vi "TLCamera Main.vi"() -> ()   [LabVIEW 2020]
uses:
  Controls/Color Balance.ctl
  Controls/Region of Interest.ctl
  Controls/Binning.ctl
  Controls/Data Rate.ctl
  Controls/Taps.ctl
  Controls/Color Modes.ctl
  Controls/Trigger Settings.ctl
  Controls/Trigger Modes.ctl
  Controls/Trigger Polarity.ctl
  Status - Main.ctl
  SubVIs/Color/Color Processor References.ctl
  SubVIs/Parameters Get & Set/Get Parameters/Get ROIAndBin.vi
  SubVIs/Parameters Get & Set/Get Parameters/Get BinXRange.vi
  SubVIs/Parameters Get & Set/Get Parameters/Get BinYRange.vi
  SubVIs/Parameters Get & Set/Get Parameters/Get CameraSensorType.vi
  SubVIs/Parameters Get & Set/Get Parameters/Get BitDepth.vi
  SubVIs/Parameters Get & Set/Get Parameters/Get SensorHeight_pixels.vi
  SubVIs/Parameters Get & Set/Get Parameters/Get SensorWidth_pixels.vi
  SubVIs/Parameters Get & Set/Get Parameters/Get ExposureTimeRange_us.vi
  SubVIs/Parameters Get & Set/Set Parameters/Set ExposureTime_us.vi
  SubVIs/Parameters Get & Set/Get Parameters/Get GainRange.vi
  SubVIs/Parameters Get & Set/Set Parameters/Set Gain.vi
  SubVIs/Parameters Get & Set/Get Parameters/Get BlackLevelRange.vi
  SubVIs/Parameters Get & Set/Set Parameters/Set BlackLevel.vi
  SubVIs/Parameters Get & Set/Set Parameters/Set ROIAndBin.vi
  SubVIs/Parameters Get & Set/Set Parameters/Set FramesPerTrigger_zeroForUnlimited.vi
  SubVIs/Parameters Get & Set/Set Parameters/Set DataRate.vi
  SubVIs/Parameters Get & Set/Set Parameters/Set Taps.vi
  C:/code/Host/Installer/Scientific Camera Interfaces/LabVIEW/32_bit/Library_X86/Thorlabs.TSI.TLCameraInterfaces.dll
  code/Host/Installer/Scientific Camera Interfaces/LabVIEW/32_bit/Library_X86/Thorlabs.TSI.TLCameraInterfaces.dll
  C:/code/Host/Installer/Scientific Camera Interfaces/LabVIEW/32_bit/Library_X86/Thorlabs.TSI.Demosaicker.dll
  code/Host/Installer/Scientific Camera Interfaces/LabVIEW/32_bit/Library_X86/Thorlabs.TSI.Demosaicker.dll
  C:/code/Host/Installer/Scientific Camera Interfaces/LabVIEW/32_bit/Library_X86/Thorlabs.TSI.ColorProcessor.dll
  code/Host/Installer/Scientific Camera Interfaces/LabVIEW/32_bit/Library_X86/Thorlabs.TSI.ColorProcessor.dll
  C:/code/Host/Installer/Scientific Camera Interfaces/LabVIEW/32_bit/Library_X86/Thorlabs.TSI.ColorInterfaces.dll
  code/Host/Installer/Scientific Camera Interfaces/LabVIEW/32_bit/Library_X86/Thorlabs.TSI.ColorInterfaces.dll
panel:
  out "event callback refnum":refnum<k27>
  out "Status":T1
  in  "Exit":bool
  out "Frame Number":u32
  out "Camera Image":picture
  in  "Camera Settings":T11={"Color Balance"={"Red Gain"=1.0, "Green Gain"=1.0, "Blue Gain"=1.0}, "Region of Interest"={"Origin - X"=0, "Origin - Y"=0, "Width"=1392, "Height"=1040}, "Binning"={"Bin - X"=1, "Bin - Y"=1}, "Frame Settings"={"Frames per Trigger\n(zero for unlimited)"=0}, "Data Rate"={"DataRate"=enum."ReadoutSpeed20MHz", "Taps"=enum."SingleTap"}, "Image Type"=enum."Standard RGB", "Trigger Settings"={"Trigger Mode"=enum."Software", "Trigger Polarity"=enum."ActiveHigh"}, "Exposure (ms)"=100.0, "Gain"=0, "Black Level"=48} {"Black Level" max=100; "Gain" max=1023; "Binning"."Bin - Y" min=1 max=16; "Binning"."Bin - X" min=1 max=16; "Color Balance"."Blue Gain" min=0 max=10 step=0.05 scale=0.0..10.0 scale format="%#_3g"; "Color Balance"."Green Gain" min=0 max=10 step=0.05 scale=0.0..10.0 scale format="%#_3g"; "Color Balance"."Red Gain" min=0 max=10 step=0.05 scale=0.0..10.0 scale format="%#_3g"}
  in  "Close Camera":bool
  in  "Open Camera":bool
  in  "Stop Camera":bool
  in  "Start Camera":bool
  in  "Refresh":bool
  in  "Camera Serial Numbers":u16(ring) items=["ENG022"]
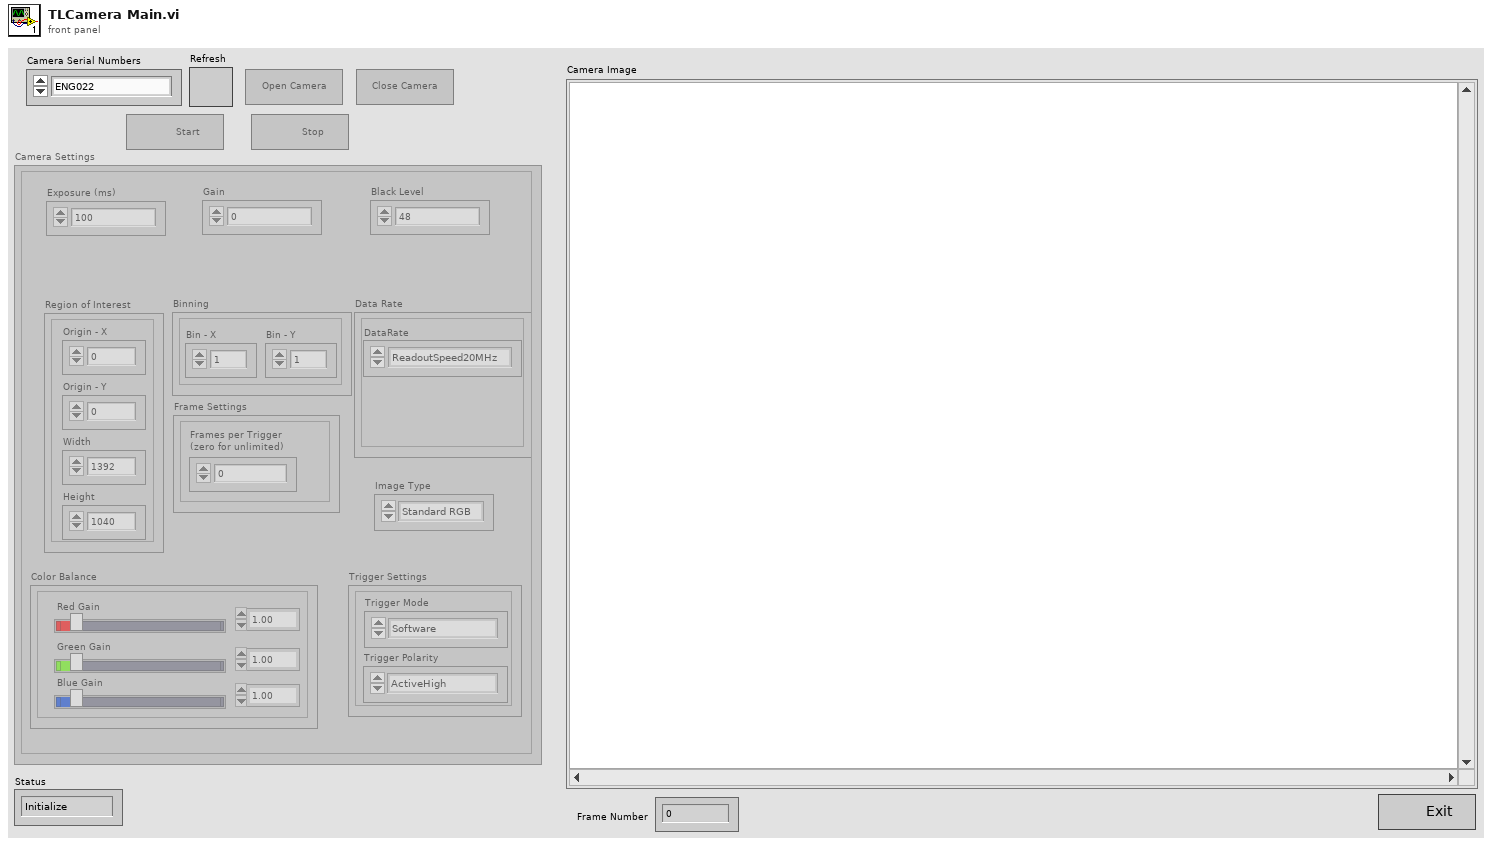
[diagram p1: front panel]
types:
  T1 = typedef "Status - Main.ctl" = enum16{"Initialize", "GUI", "Close"}
  T2 = typedef "Color Balance.ctl" = cluster{"Red Gain":sgl, "Green Gain":sgl, "Blue Gain":sgl}
  T3 = typedef "Region of Interest.ctl" = cluster{"Origin - X":u32, "Origin - Y":u32, "Width":u32, "Height":u32}
  T4 = typedef "Binning.ctl" = cluster{"Bin - X":u32, "Bin - Y":u32}
  T5 = typedef "Data Rate.ctl" = enum32{"ReadoutSpeed20MHz", "ReadoutSpeed40MHz", "FPS30", "FPS50"}
  T6 = typedef "Taps.ctl" = enum32{"SingleTap", "DualTap", "QuadTap"}
  T7 = typedef "Color Modes.ctl" = enum16{"Standard RGB", "Linear RGB", "Unprocessed"}
  T8 = typedef "Trigger Settings.ctl" = cluster{"Trigger Mode":T9, "Trigger Polarity":T10}
  T9 = typedef "Trigger Modes.ctl" = enum16{"Software", "Hardware Standard", "Bulb(PDX) Mode"}
  T10 = typedef "Trigger Polarity.ctl" = enum32{"ActiveHigh", "ActiveLow"}
  T11 = cluster{"Color Balance":T2, "Region of Interest":T3, "Binning":T4, "Frame Settings":cluster{"Frames per Trigger\n(zero for unlimited)":u32}, "Data Rate":cluster{"DataRate":T5, "Taps":T6}, "Image Type":T7, "Trigger Settings":T8, "Exposure (ms)":dbl, "Gain":u32, "Black Level":u32}
  T12 = typedef "Color Processor References.ctl" = cluster{"Demosaicker reference":refnum<k24>, "ColorProcessorSDK reference":refnum<k24>, "StandardRGBColorProcessor":refnum<k24>, "LinearRGBColorProcessor":refnum<k24>}
  T13 = enum8{"Enabled", "Disabled", "Disabled and Grayed Out"}
  T14 = cluster{"Thorlabs.TSI.TLCameraInterfaces.ITLCamera":refnum<k24>, "Frame Number":refnum<vi>, "Camera Image":refnum<vi>, "Value":T7, "Color Processor References":T12}
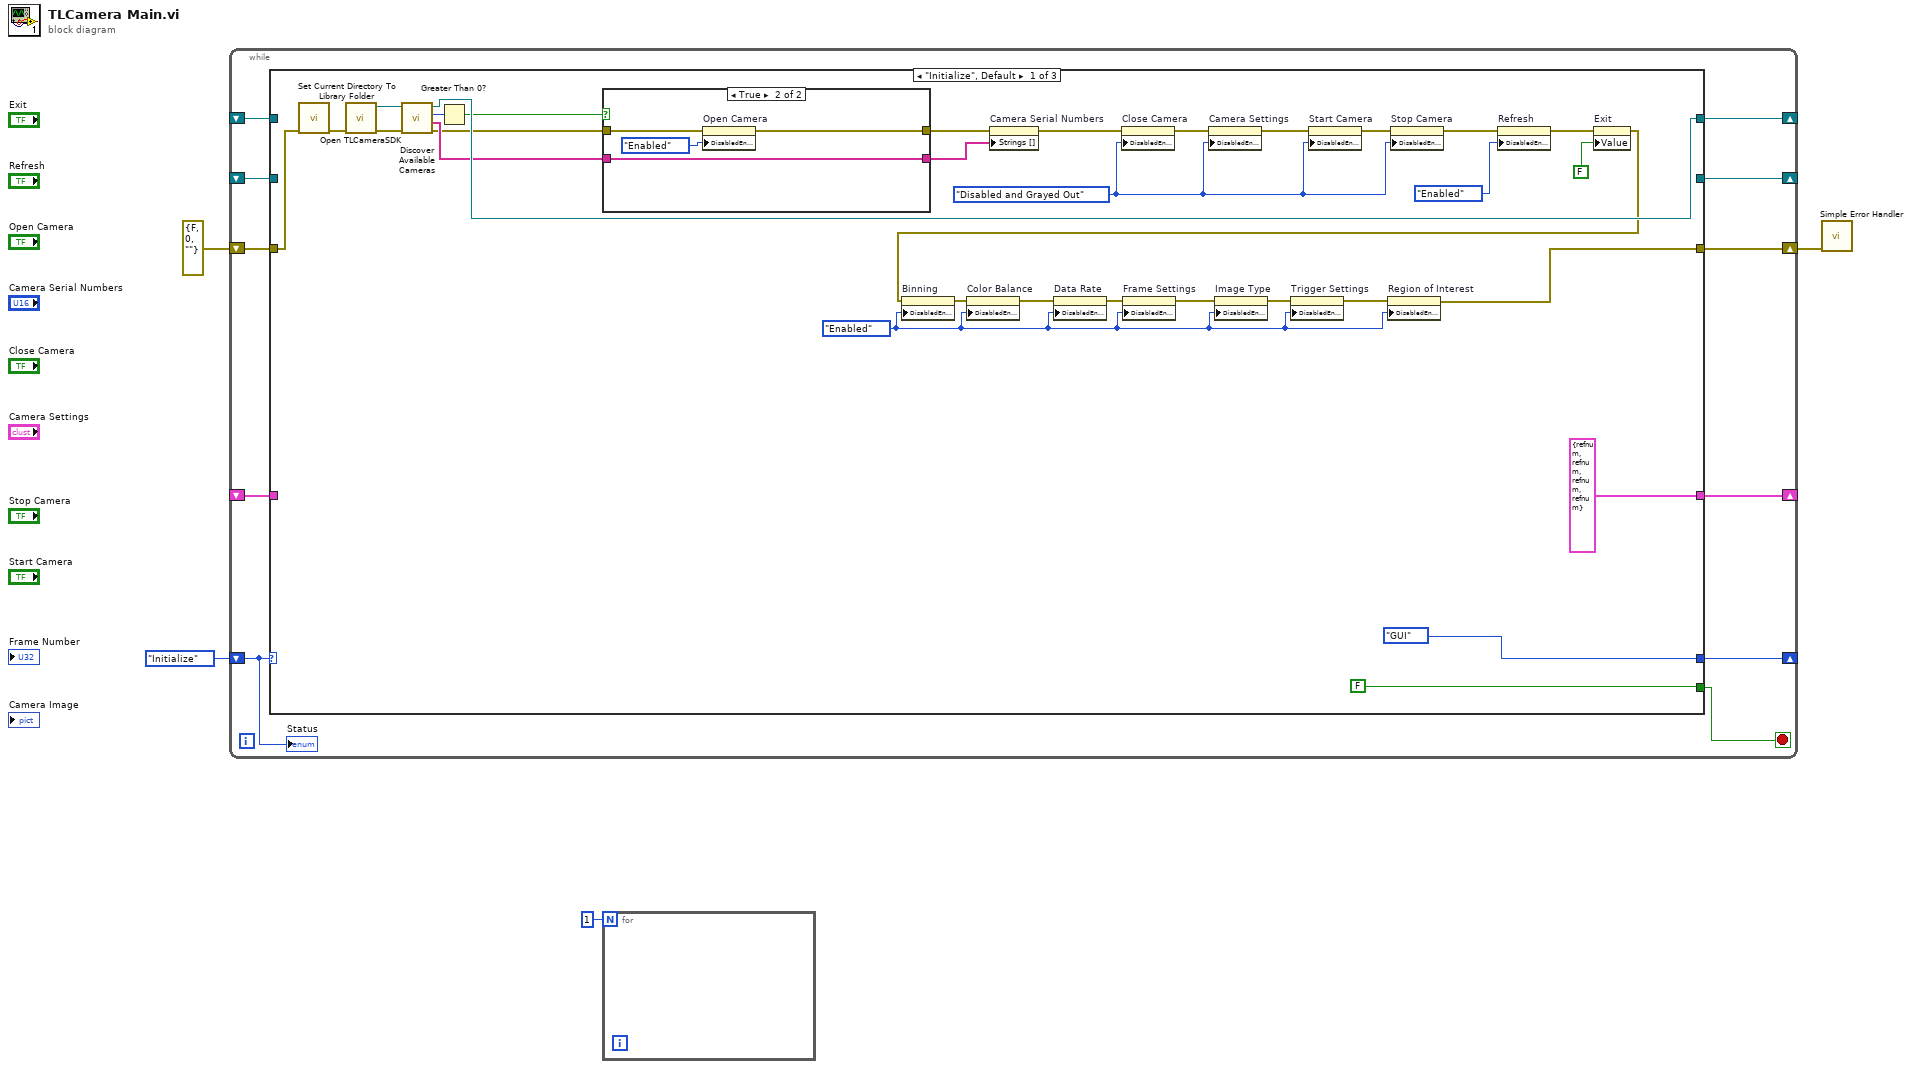
[diagram p0: block diagram]
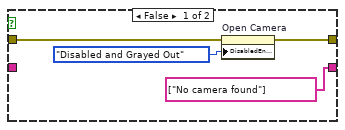
[diagram p2: hidden frame]
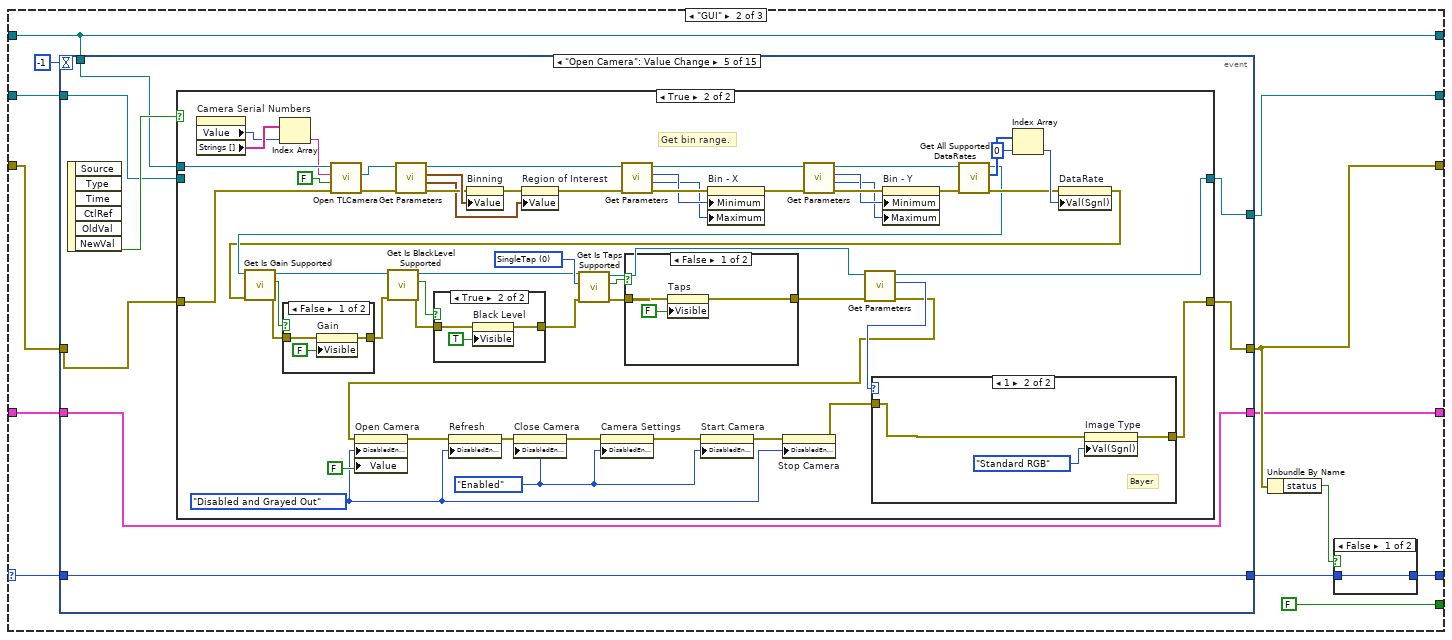
[diagram p3: hidden frame]
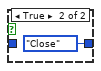
[diagram p4: hidden frame]
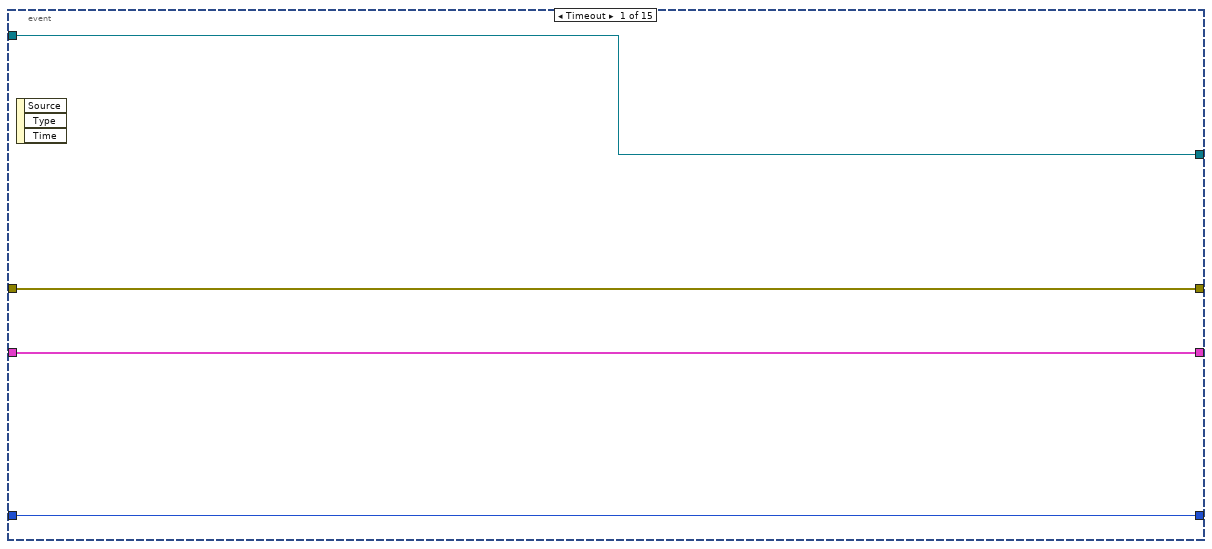
[diagram p5: hidden frame]
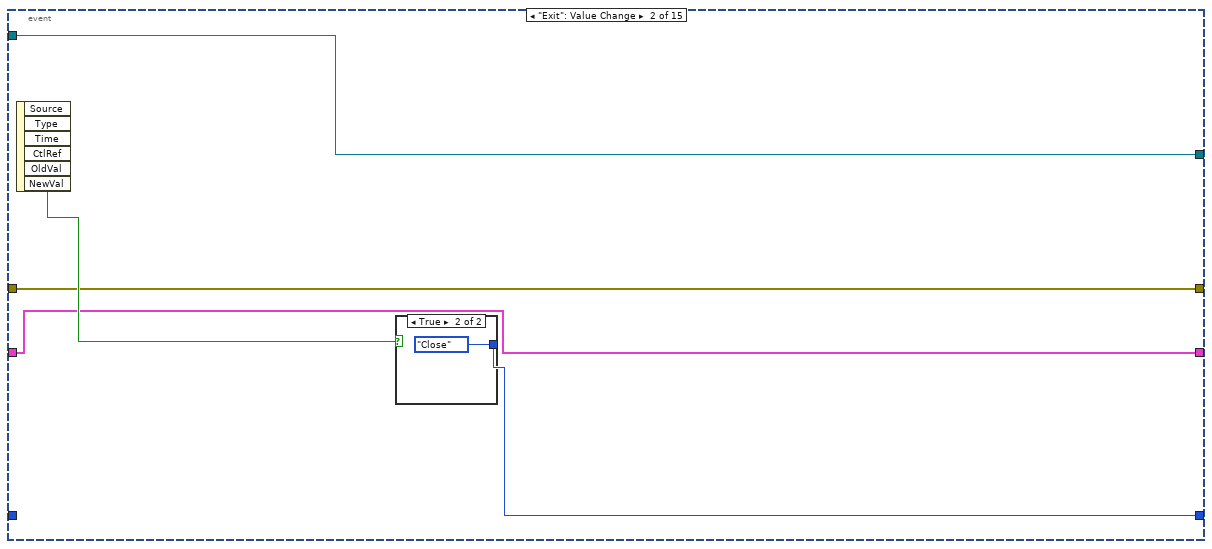
[diagram p6: hidden frame]
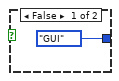
[diagram p7: hidden frame]
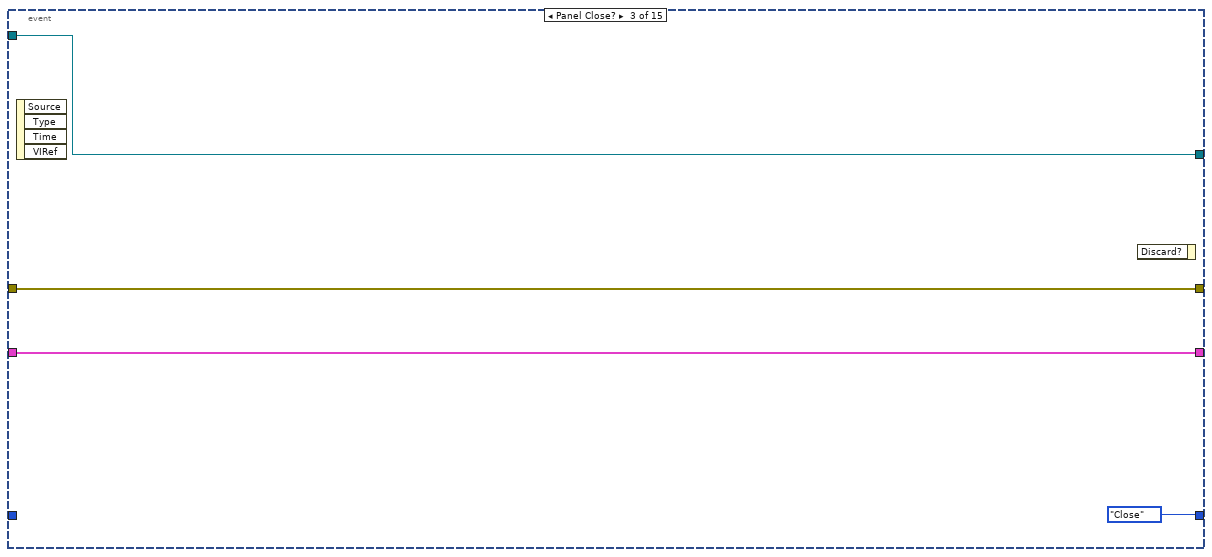
[diagram p8: hidden frame]
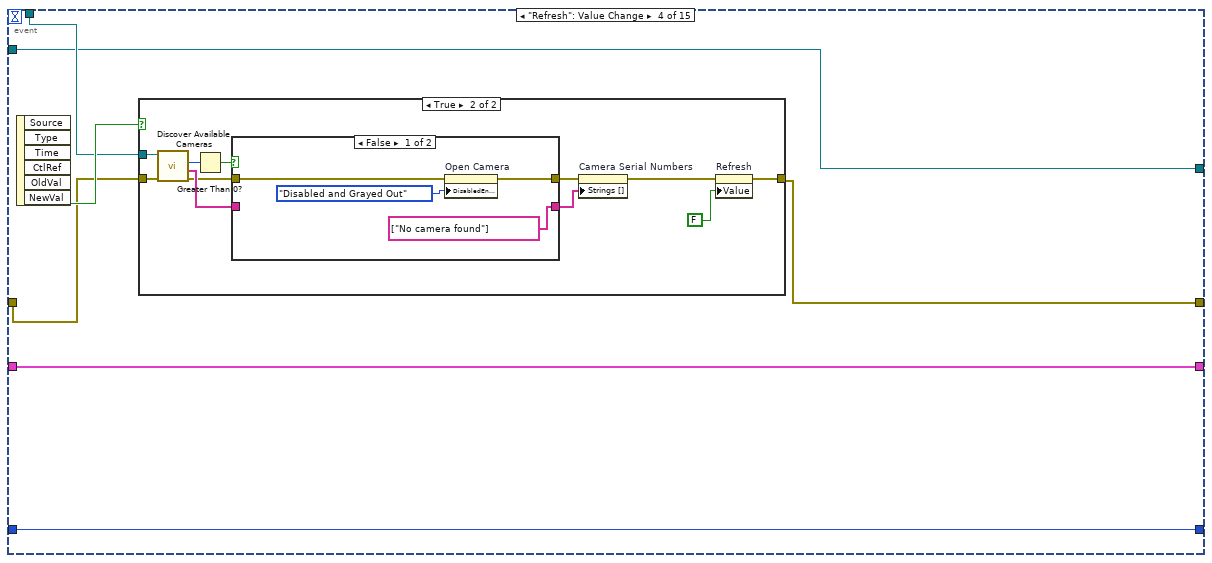
[diagram p9: hidden frame]
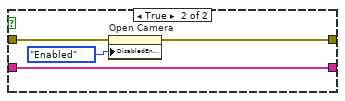
[diagram p11: hidden frame]
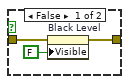
[diagram p13: hidden frame]
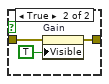
[diagram p14: hidden frame]
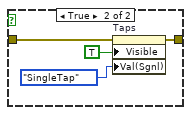
[diagram p15: hidden frame]
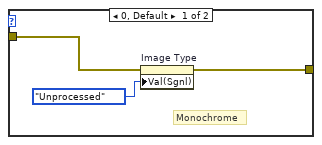
[diagram p16: hidden frame]
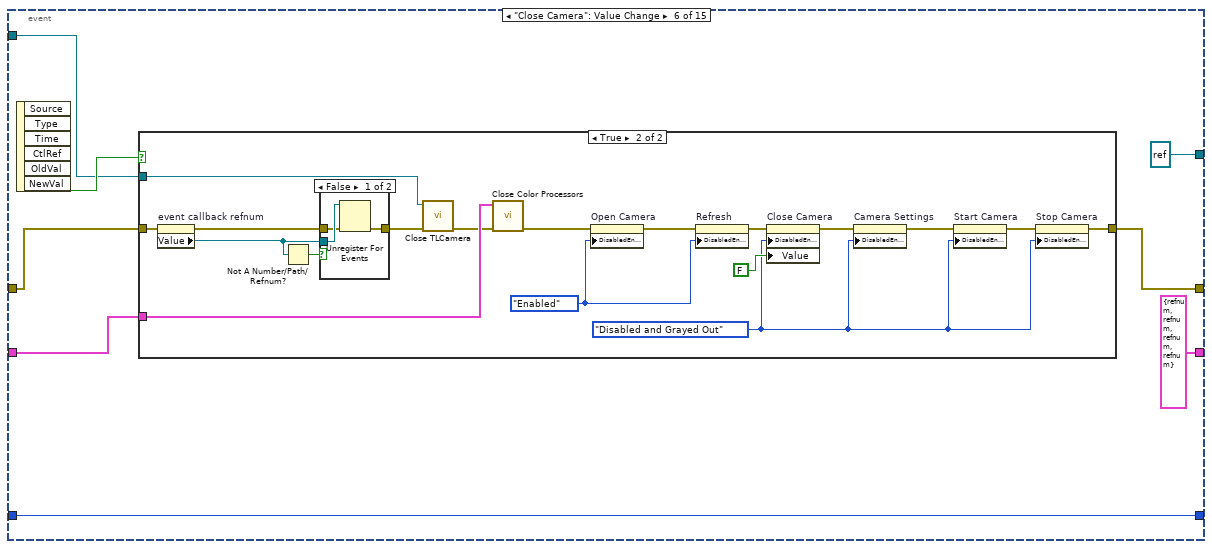
[diagram p17: hidden frame]
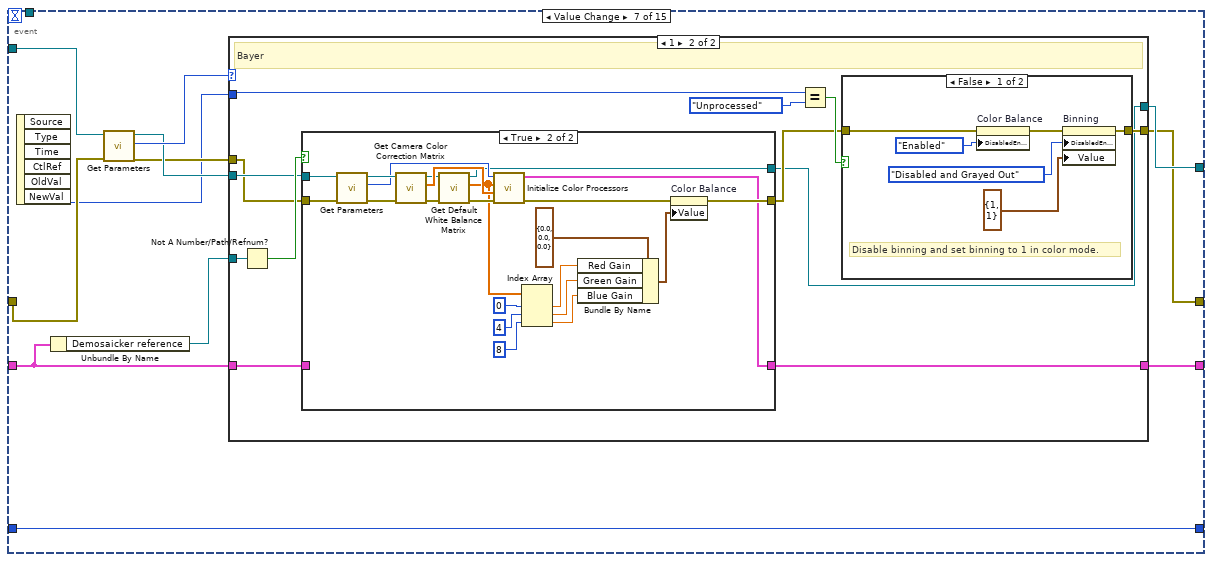
[diagram p20: hidden frame]
diagram:
  n1 = while {
    shift-right: [w8] -> _
    shift-left: Status_-_Main."Initialize" -> [w7]
    shift-right: [w15] -> _
    shift-left: _ -> [w14]
    shift-right: [w12] -> w2
    shift-left: errorcluster {"status"=FALSE, "code"=0, "source"=""} ("error in (no error)") -> [w13]
    shift-right: [w10] -> _
    shift-left: _ -> [w9]
    shift-right: [w5] -> _
    shift-left: _ -> [w6]
    stop <- w11 stop-if-true
    n2 = case shown="\"Initialize\", Default" w7 {
      selector: w7 -> [_ w66 w580]
      tunnel: [w46 w65 _] -> w15
      tunnel: w14 -> [_ w65 w582]
      tunnel: w13 -> [w18 w63 w563]
      tunnel: [w20 w62 w558] -> w12
      tunnel: [FALSE FALSE TRUE] -> w11
      tunnel: [Status_-_Main."GUI" w59 w580] -> w8
      tunnel: [_ w64 _] -> w10
      tunnel: w9 -> [_ w58 w577]
      tunnel: w6 -> [_ w57 w555]
      tunnel: [T12 {"Demosaicker reference"=refnum, "ColorProcessorSDK reference"=refnum, "StandardRGBColorProcessor"=refnum, "LinearRGBColorProcessor"=refnum} ("Color Processor References") w56 T12 {"Demosaicker reference"=refnum, "ColorProcessorSDK reference"=refnum, "StandardRGBColorProcessor"=refnum, "LinearRGBColorProcessor"=refnum} ("Color Processor References")] -> w5
      frame "Initialize", Default {
        w27 = T13."Enabled" ("Disabled")
        w36 = T13."Disabled and Grayed Out" ("Disabled")
        n3 = call "Set Current Directory To Library Folder.vi"("error in (no error)"=w18) -> ("error out"=w19:errorcluster)  [unwired: 10 in]
        n4 = call "Open TLCameraSDK.vi"("error in (no error)"=w19) -> ("error out"=w32:errorcluster, "Thorlabs.TSI.TLCameraInterfaces.ITLCameraSDK"=w31:refnum<k24>)  [unwired: 9 in]
        n5 = call "Discover Available Cameras.vi"("error in (no error)"=w32, "Thorlabs.TSI.TLCameraInterfaces.ITLCameraSDK"=w31) -> ("error out"=w42:errorcluster, "Serial Numbers"=w44:string[], "Number of Cameras"=w47:i32, "Thorlabs.TSI.TLCameraInterfaces.ITLCameraSDK"=w46:refnum<k24>)  [unwired: 6 in]
        n6 = Greater Than 0?(x=w47) -> (x > 0?=w45:bool)
        n7 = case shown="True" w45 {
          tunnel: w44 -> [_ w55]
          tunnel: [string[] ["No camera found"] ("Serial Numbers") w55] -> w43
          tunnel: w42 -> [w49 w53]
          tunnel: [w48 w52] -> w41
          frame False {
            n8 = property on="Open Camera" class="Bool (strict)"(error in=w49, "DisabledEnum"=T13."Disabled and Grayed Out" ("Disabled")) -> (error out=w48:errorcluster)  [unwired: 1 in, 1 out]
          }
          frame True {
            n9 = property on="Open Camera" class="Bool (strict)"(error in=w53, "DisabledEnum"=T13."Enabled" ("Disabled")) -> (error out=w52:errorcluster)  [unwired: 1 in, 1 out]
          }
        }
        n10 = property on="Camera Serial Numbers" class="Ring (strict)"(error in=w41, "Strings []"=w43) -> (error out=w40:errorcluster)  [unwired: 1 in, 1 out]
        n11 = property on="Close Camera" class="Bool (strict)"(error in=w40, "DisabledEnum"=w36) -> (error out=w39:errorcluster)  [unwired: 1 in, 1 out]
        n12 = property on="Camera Settings" class="Clust (strict)"(error in=w39, "DisabledEnum"=w36) -> (error out=w38:errorcluster)  [unwired: 1 in, 1 out]
        n13 = property on="Start Camera" class="Bool (strict)"(error in=w38, "DisabledEnum"=w36) -> (error out=w37:errorcluster)  [unwired: 1 in, 1 out]
        n14 = property on="Stop Camera" class="Bool (strict)"(error in=w37, "DisabledEnum"=w36) -> (error out=w30:errorcluster)  [unwired: 1 in, 1 out]
        n15 = property on="Refresh" class="Bool (strict)"(error in=w30, "DisabledEnum"=T13."Enabled" ("Disabled")) -> (error out=w29:errorcluster)  [unwired: 1 in, 1 out]
        n16 = property on="Exit" class="Bool (strict)"(error in=w29, "Value"=FALSE ("Camera Running")) -> (error out=w26:errorcluster)  [unwired: 1 in, 1 out]
        n17 = property on="Binning" class="Clust (strict)"(error in=w26, "DisabledEnum"=w27) -> (error out=w25:errorcluster)  [unwired: 1 in, 1 out]
        n18 = property on="Color Balance" class="Clust (strict)"(error in=w25, "DisabledEnum"=w27) -> (error out=w24:errorcluster)  [unwired: 1 in, 1 out]
        n19 = property on="Data Rate" class="Clust (strict)"(error in=w24, "DisabledEnum"=w27) -> (error out=w17:errorcluster)  [unwired: 1 in, 1 out]
        n20 = property on="Frame Settings" class="Clust (strict)"(error in=w17, "DisabledEnum"=w27) -> (error out=w23:errorcluster)  [unwired: 1 in, 1 out]
        n21 = property on="Image Type" class="Enum (strict)"(error in=w23, "DisabledEnum"=w27) -> (error out=w22:errorcluster)  [unwired: 1 in, 1 out]
        n22 = property on="Trigger Settings" class="Clust (strict)"(error in=w22, "DisabledEnum"=w27) -> (error out=w21:errorcluster)  [unwired: 1 in, 1 out]
        n23 = property on="Region of Interest" class="Clust (strict)"(error in=w21, "DisabledEnum"=w27) -> (error out=w20:errorcluster)  [unwired: 1 in, 1 out]
      }
      frame "GUI" {
        n24 = event shown="[4] \"Open Camera\": Value Change" {
          selector: _ -> [_ _ _ _ _ _ _ _ _ _ _ _ _ _ _]
          dyn-events: _ -> [_ _ _ _ _ _ _ _ _ _ _ _ _ _ _]
          timeout: -1 -> [_ _ _ _ _ _ _ _ _ _ _ _ _ _ _]
          tunnel: [w74 w78 Status_-_Main."Close" w88 w118 w207 w246 w317 w329 w348 w365 w396 w423 w488 w526] -> w60
          tunnel: w66 -> [w74 _ _ w88 w118 w207 w246 w317 w329 w348 w365 w396 w423 w488 w526]
          tunnel: w65 -> [_ _ _ w91 w119 _ _ _ _ _ _ _ _ _ _]
          tunnel: w63 -> [w73 w77 w84 w90 w117 w210 w245 w316 w332 w344 w367 w384 w421 w427 w529]
          tunnel: [w72 w76 w83 w87 w116 refnum<k24> refnum ("TLCamera reference") w240 w308 w320 w337 w357 w379 w424 w475 w528] -> w64
          tunnel: [w73 w77 w84 w89 w115 w209 w239 w309 w319 w336 w358 w380 w425 w472 w527] -> w62
          tunnel: w58 -> [w72 w76 w83 w87 w114 w206 w238 w307 w328 w343 w368 w379 w422 w473 w525]
          tunnel: w57 -> [w71 w75 w82 w86 w113 w204 w235 w305 w318 w334 w356 w378 w419 w438 w523]
          tunnel: [w71 w75 w82 w86 w113 T12 {"Demosaicker reference"=refnum, "ColorProcessorSDK reference"=refnum, "StandardRGBColorProcessor"=refnum, "LinearRGBColorProcessor"=refnum} ("Color Processor References") w236 w305 w318 w334 w356 w378 w419 w438 w523] -> w56
          event Timeout {
            n25 = event-data() -> ()  [unwired: 1 in, 3 out]
          }
          event "Exit": Value Change {
            n26 = event-data() -> ("NewVal"=w79:bool)  [unwired: 1 in, 5 out]
            n27 = case shown="True" w79 {
              tunnel: [Status_-_Main."GUI" Status_-_Main."Close"] -> w78
              frame False {
              }
              frame True {
              }
            }
          }
          event Panel Close? {
            n28 = event-data() -> ()  [unwired: 1 in, 4 out]
            n29 = event-data() -> ()  [unwired: 2 in, 1 out]
          }
          event "Refresh": Value Change {
            n30 = event-data() -> ("NewVal"=w92:bool)  [unwired: 1 in, 5 out]
            n31 = case shown="True" w92 {
              tunnel: w91 -> [_ w104]
              tunnel: w90 -> [w93 w103]
              tunnel: [w93 w94] -> w89
              frame False {
              }
              frame True {
                n32 = call "Discover Available Cameras.vi"("error in (no error)"=w103, "Thorlabs.TSI.TLCameraInterfaces.ITLCameraSDK"=w104) -> ("error out"=w100:errorcluster, "Serial Numbers"=w101:string[], "Number of Cameras"=w102:i32)  [unwired: 6 in, 1 out]
                n33 = Greater Than 0?(x=w102) -> (x > 0?=w97:bool)
                n34 = case shown="False" w97 {
                  tunnel: w101 -> [_ w112]
                  tunnel: [string[] ["No camera found"] ("Serial Numbers") w112] -> w99
                  tunnel: w100 -> [w106 w110]
                  tunnel: [w105 w109] -> w98
                  frame False {
                    n35 = property on="Open Camera" class="Bool (strict)"(error in=w106, "DisabledEnum"=T13."Disabled and Grayed Out" ("Disabled")) -> (error out=w105:errorcluster)  [unwired: 1 in, 1 out]
                  }
                  frame True {
                    n36 = property on="Open Camera" class="Bool (strict)"(error in=w110, "DisabledEnum"=T13."Enabled" ("Disabled")) -> (error out=w109:errorcluster)  [unwired: 1 in, 1 out]
                  }
                }
                n37 = property on="Camera Serial Numbers" class="Ring (strict)"(error in=w98, "Strings []"=w99) -> (error out=w95:errorcluster)  [unwired: 1 in, 1 out]
                n38 = property on="Refresh" class="Bool (strict)"(error in=w95, "Value"=FALSE ("Refresh")) -> (error out=w94:errorcluster)  [unwired: 1 in, 1 out]
              }
            }
          }
          event "Open Camera": Value Change {
            n39 = event-data() -> ("NewVal"=w120:bool)  [unwired: 1 in, 5 out]
            n40 = case shown="True" w120 {
              tunnel: w119 -> [_ w178]
              tunnel: w117 -> [w121 w146]
              tunnel: [w122 w124] -> w116
              tunnel: w114 -> [w122 _]
              tunnel: [w121 w147] -> w115
              frame False {
              }
              frame True {
                w145 = 0 items=["SingleTap", "DualTap", "QuadTap"] ("Taps")
                w165 = T13."Enabled" ("Disabled")
                w166 = T13."Disabled and Grayed Out" ("Disabled")
                # "Get bin range."
                n41 = property on="Camera Serial Numbers" class="Ring (strict)"() -> ("Value"=w176:u16, "Strings []"=w177:string[])  [unwired: 2 in, 2 out]
                n42 = Index Array(array=w177, index=w176) -> (element=w175:string)
                n43 = call "Open TLCamera.vi"("error in (no error)"=w146, "isDiagnosticsMessagesEnabled"=FALSE, "Camera serial number"=w175, "Thorlabs.TSI.TLCameraInterfaces.ITLCameraSDK"=w178) -> ("error out"=w163:errorcluster, "Thorlabs.TSI.TLCameraInterfaces.ITLCamera"=w162:refnum<k24>)  [unwired: 5 in, 1 out]
                n44 = call-poly "Get Parameters.vi"("error in (no error)"=w163, "Thorlabs.TSI.TLCameraInterfaces.ITLCamera"=w162) -> ("error out"=w160:errorcluster, "Region of Interest"=w159:T3, "Binning"=w161:T4, "Thorlabs.TSI.TLCameraInterfaces.ITLCamera"=w148:refnum<k24>)  [unwired: 6 in]
                n45 = property on="Binning" class="Clust (strict)"(error in=w160, "Value"=w161) -> (error out=w158:errorcluster)  [unwired: 1 in, 1 out]
                n46 = property on="Region of Interest" class="Clust (strict)"(error in=w158, "Value"=w159) -> (error out=w149:errorcluster)  [unwired: 1 in, 1 out]
                n47 = call-poly "Get Parameters.vi"("error in (no error)"=w149, "Thorlabs.TSI.TLCameraInterfaces.ITLCamera"=w148) -> ("error out"=w157:errorcluster, "Maximum"=w155:u32, "Minimum"=w156:u32, "Thorlabs.TSI.TLCameraInterfaces.ITLCamera"=w153:refnum<k24>)  [unwired: 6 in]
                n48 = property on="Bin - X" class="DigNum (strict)"(error in=w157, "Minimum"=w156, "Maximum"=w155) -> (error out=w154:errorcluster)  [unwired: 1 in, 1 out]
                n49 = call-poly "Get Parameters.vi"("error in (no error)"=w154, "Thorlabs.TSI.TLCameraInterfaces.ITLCamera"=w153) -> ("error out"=w152:errorcluster, "Maximum"=w150:u32, "Minimum"=w151:u32, "Thorlabs.TSI.TLCameraInterfaces.ITLCamera"=w144:refnum<k24>)  [unwired: 6 in]
                n50 = property on="Bin - Y" class="DigNum (strict)"(error in=w152, "Minimum"=w151, "Maximum"=w150) -> (error out=w143:errorcluster)  [unwired: 1 in, 1 out]
                n51 = call "Get All Supported DataRates.vi"("error in (no error)"=w143, "Thorlabs.TSI.TLCameraInterfaces.ITLCamera"=w144) -> ("error out"=w139:errorcluster, "Supported DataRates"=w142:i32[], "Thorlabs.TSI.TLCameraInterfaces.ITLCamera"=w134:refnum<k24>)  [unwired: 7 in]
                n52 = Index Array(array=w142, index=0) -> (element=w140:i32)
                n53 = property on="DataRate" class="Enum (strict)"(error in=w139, "Val(Sgnl)"=w140) -> (error out=w133:errorcluster)  [unwired: 1 in, 1 out]
                n54 = call "Get Is Gain Supported.vi"("error in (no error)"=w133, "Thorlabs.TSI.TLCameraInterfaces.ITLCamera"=w134) -> ("error out"=w131:errorcluster, "Is Gain Supported?"=w132:bool, "Thorlabs.TSI.TLCameraInterfaces.ITLCamera"=w129:refnum<k24>)  [unwired: 7 in]
                n55 = case shown="False" w132 {
                  tunnel: w131 -> [w186 w190]
                  tunnel: [w185 w188] -> w130
                  frame False {
                    n56 = property on="Gain" class="DigNum (strict)"(error in=w186, "Visible"=FALSE) -> (error out=w185:errorcluster)  [unwired: 1 in, 1 out]
                  }
                  frame True {
                    n57 = property on="Gain" class="DigNum (strict)"(error in=w190, "Visible"=TRUE) -> (error out=w188:errorcluster)  [unwired: 1 in, 1 out]
                  }
                }
                n58 = call "Get Is BlackLevel Supported.vi"("error in (no error)"=w130, "Thorlabs.TSI.TLCameraInterfaces.ITLCamera"=w129) -> ("error out"=w127:errorcluster, "Is BlackLevel Supported?"=w128:bool, "Thorlabs.TSI.TLCameraInterfaces.ITLCamera"=w125:refnum<k24>)  [unwired: 7 in]
                n59 = case shown="True" w128 {
                  tunnel: w127 -> [w180 w184]
                  tunnel: [w179 w182] -> w126
                  frame False {
                    n60 = property on="Black Level" class="DigNum (strict)"(error in=w180, "Visible"=FALSE) -> (error out=w179:errorcluster)  [unwired: 1 in, 1 out]
                  }
                  frame True {
                    n61 = property on="Black Level" class="DigNum (strict)"(error in=w184, "Visible"=TRUE) -> (error out=w182:errorcluster)  [unwired: 1 in, 1 out]
                  }
                }
                n62 = call "Get Is Taps Supported.vi"("error in (no error)"=w126, "Taps"=w145, "Thorlabs.TSI.TLCameraInterfaces.ITLCamera"=w125) -> ("error out"=w137:errorcluster, "Is Taps Supported"=w138:bool, "Thorlabs.TSI.TLCameraInterfaces.ITLCamera"=w136:refnum<k24>)  [unwired: 6 in]
                n63 = case shown="False" w138 {
                  tunnel: w137 -> [w192 w197]
                  tunnel: [w191 w196] -> w135
                  frame False {
                    n64 = property on="Taps" class="Enum (strict)"(error in=w192, "Visible"=FALSE) -> (error out=w191:errorcluster)  [unwired: 1 in, 1 out]
                  }
                  frame True {
                    n65 = property on="Taps" class="Enum (strict)"(error in=w197, "Visible"=TRUE, "Val(Sgnl)"=Taps."SingleTap" ("Value (Signaling)")) -> (error out=w196:errorcluster)  [unwired: 1 in, 1 out]
                  }
                }
                n66 = call-poly "Get Parameters.vi"("error in (no error)"=w135, "Thorlabs.TSI.TLCameraInterfaces.ITLCamera"=w136) -> ("error out"=w123:errorcluster, "CameraSensorType"=w164:i32, "Thorlabs.TSI.TLCameraInterfaces.ITLCamera"=w124:refnum<k24>)  [unwired: 7 in]
                n67 = property on="Open Camera" class="Bool (strict)"(error in=w123, "DisabledEnum"=w166, "Value"=FALSE ("Open Camera")) -> (error out=w171:errorcluster)  [unwired: 1 in, 1 out]
                n68 = property on="Refresh" class="Bool (strict)"(error in=w171, "DisabledEnum"=w166) -> (error out=w170:errorcluster)  [unwired: 1 in, 1 out]
                n69 = property on="Close Camera" class="Bool (strict)"(error in=w170, "DisabledEnum"=w165) -> (error out=w172:errorcluster)  [unwired: 1 in, 1 out]
                n70 = property on="Camera Settings" class="Clust (strict)"(error in=w172, "DisabledEnum"=w165) -> (error out=w169:errorcluster)  [unwired: 1 in, 1 out]
                n71 = property on="Start Camera" class="Bool (strict)"(error in=w169, "DisabledEnum"=w165) -> (error out=w168:errorcluster)  [unwired: 1 in, 1 out]
                n72 = property on="Stop Camera" class="Bool (strict)"(error in=w168, "DisabledEnum"=w166) -> (error out=w167:errorcluster)  [unwired: 1 in, 1 out]
                n73 = case shown="1" w164 {
                  tunnel: w167 -> [w198 w201]
                  tunnel: [w200 w203] -> w147
                  frame 0, Default {
                    # "Monochrome"
                    n74 = property on="Image Type" class="Enum (strict)"(error in=w198, "Val(Sgnl)"=Color_Modes."Unprocessed" ("Value")) -> (error out=w200:errorcluster)  [unwired: 1 in, 1 out]
                  }
                  frame 1 {
                    # "Bayer"
                    n75 = property on="Image Type" class="Enum (strict)"(error in=w201, "Val(Sgnl)"=Color_Modes."Standard RGB" ("Value")) -> (error out=w203:errorcluster)  [unwired: 1 in, 1 out]
                  }
                }
              }
            }
          }
          event "Close Camera": Value Change {
            n76 = event-data() -> ("NewVal"=w211:bool)  [unwired: 1 in, 5 out]
            n77 = case shown="True" w211 {
              tunnel: w206 -> [_ w230]
              tunnel: w210 -> [w212 w219]
              tunnel: [w212 w223] -> w209
              tunnel: w204 -> [_ w215]
              frame False {
              }
              frame True {
                w216 = T13."Disabled and Grayed Out" ("Disabled")
                w224 = T13."Enabled" ("Disabled")
                n78 = property on="event callback refnum" class="Ref (strict)"(error in=w219) -> (error out=w220:errorcluster, "Value"=w221:refnum<k27>)  [unwired: 1 in, 1 out]
                n79 = Not A Number/Path/Refnum?(number/path/refnum=w221) -> (NaN/Path/Refnum?=w222:bool)
                n80 = case shown="False" w222 {
                  tunnel: w221 -> [w233 _]
                  tunnel: w220 -> [w232 w234]
                  tunnel: [w231 w234] -> w218
                  frame False {
                    n81 = Unregister For Events(event registration refnum=w233, error in=w232) -> (error out=w231:errorcluster)
                  }
                  frame True {
                  }
                }
                n82 = call "Close TLCamera.vi"("error in (no error)"=w218, "Thorlabs.TSI.TLCameraInterfaces.ITLCamera"=w230) -> ("error out"=w214:errorcluster)  [unwired: 9 in]
                n83 = call "Close Color Processors.vi"("error in (no error)"=w214, "Color Processor References"=w215) -> ("error out"=w213:errorcluster)  [unwired: 9 in]
                n84 = property on="Open Camera" class="Bool (strict)"(error in=w213, "DisabledEnum"=w224) -> (error out=w226:errorcluster)  [unwired: 1 in, 1 out]
                n85 = property on="Refresh" class="Bool (strict)"(error in=w226, "DisabledEnum"=w224) -> (error out=w225:errorcluster)  [unwired: 1 in, 1 out]
                n86 = property on="Close Camera" class="Bool (strict)"(error in=w225, "DisabledEnum"=w216, "Value"=FALSE ("Close Camera")) -> (error out=w229:errorcluster)  [unwired: 1 in, 1 out]
                n87 = property on="Camera Settings" class="Clust (strict)"(error in=w229, "DisabledEnum"=w216) -> (error out=w217:errorcluster)  [unwired: 1 in, 1 out]
                n88 = property on="Start Camera" class="Bool (strict)"(error in=w217, "DisabledEnum"=w216) -> (error out=w227:errorcluster)  [unwired: 1 in, 1 out]
                n89 = property on="Stop Camera" class="Bool (strict)"(error in=w227, "DisabledEnum"=w216) -> (error out=w223:errorcluster)  [unwired: 1 in, 1 out]
              }
            }
          }
          event Value Change {
            n90 = event-data() -> ("NewVal"=w241:T7)  [unwired: 1 in, 5 out]
            n91 = Unbundle By Name(w235) -> ("Demosaicker reference"=w237:refnum<k24>)
            n92 = call-poly "Get Parameters.vi"("error in (no error)"=w245, "Thorlabs.TSI.TLCameraInterfaces.ITLCamera"=w238) -> ("error out"=w242:errorcluster, "CameraSensorType"=w244:i32, "Thorlabs.TSI.TLCameraInterfaces.ITLCamera"=w243:refnum<k24>)  [unwired: 7 in]
            n93 = case shown="1" w244 {
              tunnel: w243 -> [w249 w262]
              tunnel: w242 -> [w252 w261]
              tunnel: w241 -> [_ w265]
              tunnel: [w249 w259] -> w240
              tunnel: [w253 w266] -> w239
              tunnel: w237 -> [_ w264]
              tunnel: [w247 w257] -> w236
              tunnel: w235 -> [w247 w258]
              frame 0, Default {
                # "Monochrome"
                n94 = property on="Image Type" class="Enum (strict)"(error in=w252, "Value"=Color_Modes."Unprocessed") -> (error out=w250:errorcluster)  [unwired: 1 in, 1 out]
                n95 = property on="Binning" class="Clust (strict)"(error in=w250, "DisabledEnum"=T13."Enabled" ("Disabled"), "Value"=T4 {"Bin - X"=1, "Bin - Y"=1}) -> (error out=w254:errorcluster)  [unwired: 1 in, 1 out]
                n96 = property on="Color Balance" class="Clust (strict)"(error in=w254, "DisabledEnum"=T13."Disabled and Grayed Out" ("Disabled")) -> (error out=w253:errorcluster)  [unwired: 1 in, 1 out]
              }
              frame 1 {
                # "Bayer"
                n97 = Not A Number/Path/Refnum?(number/path/refnum=w264) -> (NaN/Path/Refnum?=w263:bool)
                n98 = case shown="True" w263 {
                  tunnel: w262 -> [w270 w289]
                  tunnel: w261 -> [w271 w290]
                  tunnel: [w271 w274] -> w260
                  tunnel: [w270 w273] -> w259
                  tunnel: w258 -> [w269 _]
                  tunnel: [w269 w272] -> w257
                  frame False {
                  }
                  frame True {
                    n99 = call-poly "Get Parameters.vi"("error in (no error)"=w290, "Thorlabs.TSI.TLCameraInterfaces.ITLCamera"=w289) -> ("error out"=w287:errorcluster, "BitDepth"=w286:u32, "Thorlabs.TSI.TLCameraInterfaces.ITLCamera"=w288:refnum<k24>)  [unwired: 7 in]
                    n100 = call "Get Camera Color Correction Matrix.vi"("error in (no error)"=w287, "Thorlabs.TSI.TLCameraInterfaces.ITLCamera"=w288) -> ("error out"=w292:errorcluster, "Camera Color Correction Matrix"=w293:sgl[], "Thorlabs.TSI.TLCameraInterfaces.ITLCamera"=w291:refnum<k24>)  [unwired: 7 in]
                    n101 = call "Get Default White Balance Matrix.vi"("error in (no error)"=w292, "Thorlabs.TSI.TLCameraInterfaces.ITLCamera"=w291) -> ("error out"=w285:errorcluster, "Default White Balance Matrix"=w284:sgl[], "Thorlabs.TSI.TLCameraInterfaces.ITLCamera"=w273:refnum<k24>)  [unwired: 7 in]
                    n102 = call "Initialize Color Processors.vi"("error in (no error)"=w285, "Camera Color Correction Matrix"=w293, "White Balance Matrix"=w284, "BitDepth"=w286) -> ("error out"=w275:errorcluster, "Color Processor References"=w272:T12)  [unwired: 6 in]
                    n103 = Index Array(array=w284, index #1=0 ("index"), index #2=4 ("index"), index #3=8 ("index")) -> (element #1=w278:sgl, element #2=w277:sgl, element #3=w276:sgl)
                    n104 = Bundle By Name(cluster=T2 {"Red Gain"=0.0, "Green Gain"=0.0, "Blue Gain"=0.0} ("Value"), "Red Gain"=w278, "Green Gain"=w277, "Blue Gain"=w276) -> (w280:T2)
                    n105 = property on="Color Balance" class="Clust (strict)"(error in=w275, "Value"=w280) -> (error out=w274:errorcluster)  [unwired: 1 in, 1 out]
                  }
                }
                n106 = Equal?(x=w265, y=Color_Modes."Unprocessed") -> (x = y?=w267:bool)
                n107 = case shown="False" w267 {
                  tunnel: w260 -> [w294 w300]
                  tunnel: [w295 w301] -> w266
                  frame False {
                    # "Disable binning and set binning to 1 in color mode."
                    n108 = property on="Color Balance" class="Clust (strict)"(error in=w294, "DisabledEnum"=T13."Enabled" ("Disabled")) -> (error out=w299:errorcluster)  [unwired: 1 in, 1 out]
                    n109 = property on="Binning" class="Clust (strict)"(error in=w299, "DisabledEnum"=T13."Disabled and Grayed Out" ("Disabled"), "Value"=T4 {"Bin - X"=1, "Bin - Y"=1} ("Value (Signaling)")) -> (error out=w295:errorcluster)  [unwired: 1 in, 1 out]
                  }
                  frame True {
                    # "Enable binning and disable color balance"
                    n110 = property on="Binning" class="Clust (strict)"(error in=w300, "DisabledEnum"=T13."Enabled" ("Disabled")) -> (error out=w304:errorcluster)  [unwired: 1 in, 1 out]
                    n111 = property on="Color Balance" class="Clust (strict)"(error in=w304, "DisabledEnum"=T13."Disabled and Grayed Out" ("Disabled")) -> (error out=w301:errorcluster)  [unwired: 1 in, 1 out]
                  }
                }
              }
            }
          }
          event Value Change {
            n112 = event-data() -> ("NewVal"=w306:T3)  [unwired: 1 in, 5 out]
            n113 = call-poly "Get Parameters.vi"("error in (no error)"=w316, "Thorlabs.TSI.TLCameraInterfaces.ITLCamera"=w307) -> ("error out"=w314:errorcluster, "SensorHeight_pixels"=w312:u32, "Thorlabs.TSI.TLCameraInterfaces.ITLCamera"=w315:refnum<k24>)  [unwired: 7 in]
            n114 = call-poly "Get Parameters.vi"("error in (no error)"=w314, "Thorlabs.TSI.TLCameraInterfaces.ITLCamera"=w315) -> ("error out"=w310:errorcluster, "SensorWidth_pixels"=w313:u32, "Thorlabs.TSI.TLCameraInterfaces.ITLCamera"=w308:refnum<k24>)  [unwired: 7 in]
            n115 = call "Validate ROI.vi"("ROI in"=w306, "SensorHeight_pixels"=w312, "SensorWidth_pixels"=w313) -> ("ROI out"=w311:T3)  [unwired: 8 in]
            n116 = property on="Region of Interest" class="Clust (strict)"(error in=w310, "Value"=w311) -> (error out=w309:errorcluster)  [unwired: 1 in, 1 out]
          }
          event "Camera Settings.Exposure (ms)": Value Change {
            n117 = event-data() -> ("NewVal"=w327:dbl)  [unwired: 1 in, 5 out]
            n118 = call-poly "Get Parameters.vi"("error in (no error)"=w332, "Thorlabs.TSI.TLCameraInterfaces.ITLCamera"=w328) -> ("error out"=w324:errorcluster, "Maximum"=w330:u32, "Thorlabs.TSI.TLCameraInterfaces.ITLCamera"=w323:refnum<k24>)  [unwired: 6 in, 1 out]
            n119 = Multiply(x=1000.0, y=w327) -> (x*y=w331:dbl)
            n120 = Max & Min(x=w330, y=w331) -> (min(x,y)=w321:dbl)  [unwired: 1 out]
            n121 = Divide(x=w321, y=1000.0) -> (x/y=w325:dbl)
            n122 = property on="Exposure (ms)" class="DigNum (strict)"(error in=w324, "Value"=w325) -> (error out=w322:errorcluster)  [unwired: 1 in, 1 out]
            n123 = call-poly "Set Parameters.vi"("error in (no error)"=w322, "ExposureTime_us"=w321, "Thorlabs.TSI.TLCameraInterfaces.ITLCamera"=w323) -> ("error out"=w319:errorcluster, "Thorlabs.TSI.TLCameraInterfaces.ITLCamera"=w320:refnum<k24>)  [unwired: 7 in]
          }
          event "Camera Settings.Gain": Value Change {
            n124 = event-data() -> ("NewVal"=w345:u32)  [unwired: 1 in, 5 out]
            n125 = call-poly "Get Parameters.vi"("error in (no error)"=w344, "Thorlabs.TSI.TLCameraInterfaces.ITLCamera"=w343) -> ("error out"=w346:errorcluster, "Maximum"=w347:u32, "Thorlabs.TSI.TLCameraInterfaces.ITLCamera"=w342:refnum<k24>)  [unwired: 6 in, 1 out]
            n126 = Max & Min(x=w347, y=w345) -> (min(x,y)=w335:u32)  [unwired: 1 out]
            n127 = property on="Gain" class="DigNum (strict)"(error in=w346, "Value"=w335) -> (error out=w341:errorcluster)  [unwired: 1 in, 1 out]
            n128 = call "Get Is Gain Supported.vi"("error in (no error)"=w341, "Thorlabs.TSI.TLCameraInterfaces.ITLCamera"=w342) -> ("error out"=w338:errorcluster, "Is Gain Supported?"=w340:bool, "Thorlabs.TSI.TLCameraInterfaces.ITLCamera"=w339:refnum<k24>)  [unwired: 7 in]
            n129 = case shown="True" w340 {
              tunnel: w339 -> [w350 w355]
              tunnel: w338 -> [w349 w354]
              tunnel: [w350 w353] -> w337
              tunnel: [w349 w352] -> w336
              tunnel: w335 -> [_ w351]
              frame False {
              }
              frame True {
                n130 = call-poly "Set Parameters.vi"("error in (no error)"=w354, "Gain"=w351, "Thorlabs.TSI.TLCameraInterfaces.ITLCamera"=w355) -> ("error out"=w352:errorcluster, "Thorlabs.TSI.TLCameraInterfaces.ITLCamera"=w353:refnum<k24>)  [unwired: 7 in]
              }
            }
          }
          event "Camera Settings.Black Level": Value Change {
            n131 = event-data() -> ("NewVal"=w366:u32)  [unwired: 1 in, 5 out]
            n132 = call-poly "Get Parameters.vi"("error in (no error)"=w367, "Thorlabs.TSI.TLCameraInterfaces.ITLCamera"=w368) -> ("error out"=w369:errorcluster, "Maximum"=w370:u32, "Thorlabs.TSI.TLCameraInterfaces.ITLCamera"=w364:refnum<k24>)  [unwired: 6 in, 1 out]
            n133 = Max & Min(x=w370, y=w366) -> (min(x,y)=w359:u32)  [unwired: 1 out]
            n134 = property on="Black Level" class="DigNum (strict)"(error in=w369, "Value"=w359) -> (error out=w363:errorcluster)  [unwired: 1 in, 1 out]
            n135 = call "Get Is BlackLevel Supported.vi"("error in (no error)"=w363, "Thorlabs.TSI.TLCameraInterfaces.ITLCamera"=w364) -> ("error out"=w360:errorcluster, "Is BlackLevel Supported?"=w362:bool, "Thorlabs.TSI.TLCameraInterfaces.ITLCamera"=w361:refnum<k24>)  [unwired: 7 in]
            n136 = case shown="False" w362 {
              tunnel: w361 -> [w372 w377]
              tunnel: w360 -> [w371 w376]
              tunnel: w359 -> [_ w375]
              tunnel: [w371 w374] -> w358
              tunnel: [w372 w373] -> w357
              frame False {
              }
              frame True {
                n137 = call-poly "Set Parameters.vi"("error in (no error)"=w376, "BlackLevel"=w375, "Thorlabs.TSI.TLCameraInterfaces.ITLCamera"=w377) -> ("error out"=w374:errorcluster, "Thorlabs.TSI.TLCameraInterfaces.ITLCamera"=w373:refnum<k24>)  [unwired: 7 in]
              }
            }
          }
          event "Camera Settings.Data Rate": Value Change {
            n138 = event-data() -> ()  [unwired: 1 in, 6 out]
            n139 = property on="DataRate" class="Enum (strict)"(error in=w384) -> (error out=w385:errorcluster, "NumItems"=w395:u32, "Value"=w393:T5)  [unwired: 1 in, 1 out]
            n140 = property on="Taps" class="Enum (strict)"(error in=w384) -> (error out=w383:errorcluster, "NumItems"=w390:u32, "Value"=w388:T6)  [unwired: 1 in, 1 out]
            n141 = Initialize Array(w393) -> (w394:T5[])  [unwired: 1 in]
            n142 = Initialize Array(w388) -> (w389:T6[])  [unwired: 1 in]
            n143 = for {
              N: w395 -> [_]
              tunnel: w379 -> [w414]
              shift-right: [w410] -> w392
              shift-left: w394 -> [w411]
              shift-right: [w408] -> w391
              shift-left: w385 -> [w413]
              i -> [w409]
              n144 = call "Get Is DataRate Supported.vi"("error in (no error)"=w413, "Data Rate"=w409, "Thorlabs.TSI.TLCameraInterfaces.ITLCamera"=w414) -> ("error out"=w408:errorcluster, "Is DataRate Supported"=w412:bool)  [unwired: 6 in, 1 out]
              n145 = case shown="False" w412 {
                tunnel: w411 -> [w417 w418]
                tunnel: [w415 w418] -> w410
                tunnel: w409 -> [w416 _]
                frame False {
                  n146 = Build Array (concatenate)(w417, w416) -> (w415:u32[])
                }
                frame True {
                }
              }
            }
            n147 = for {
              N: w390 -> [_]
              tunnel: w379 -> [w403]
              shift-right: [w399] -> w387
              shift-left: w389 -> [w400]
              shift-right: [w397] -> w386
              shift-left: w383 -> [w402]
              i -> [w398]
              n148 = call "Get Is Taps Supported.vi"("error in (no error)"=w402, "Taps"=w398, "Thorlabs.TSI.TLCameraInterfaces.ITLCamera"=w403) -> ("error out"=w397:errorcluster, "Is Taps Supported"=w401:bool)  [unwired: 6 in, 1 out]
              n149 = case shown="False" w401 {
                tunnel: w400 -> [w406 w407]
                tunnel: [w404 w407] -> w399
                tunnel: w398 -> [w405 _]
                frame False {
                  n150 = Build Array (concatenate)(w406, w405) -> (w404:u32[])
                }
                frame True {
                }
              }
            }
            n151 = property on="DataRate" class="Enum (strict)"(error in=w391, "Disabled Items []"=w392) -> (error out=w382:errorcluster)  [unwired: 1 in, 1 out]
            n152 = property on="Taps" class="Enum (strict)"(error in=w386, "Disabled Items []"=w387) -> (error out=w381:errorcluster)  [unwired: 1 in, 1 out]
            n153 = Merge Errors(w382, w381) -> (w380:errorcluster)
          }
          event Value Change {
            n154 = event-data() -> ("NewVal"=w420:T2)  [unwired: 1 in, 5 out]
            n155 = call "Set Color Balance.vi"("error in (no error)"=w421, "NewVal"=w420, "Color Processor References"=w419, "Thorlabs.TSI.TLCameraInterfaces.ITLCamera"=w422) -> ("error out"=w425:errorcluster, "Thorlabs.TSI.TLCameraInterfaces.ITLCamera"=w424:refnum<k24>)  [unwired: 6 in]
          }
          event "Start Camera": Value Change {
            w428 = T13."Disabled and Grayed Out" ("Disabled")
            n156 = event-data() -> ()  [unwired: 1 in, 6 out]
            n157 = property on="Start Camera" class="Bool (strict)"(error in=w427, "DisabledEnum"=w428, "Value"=FALSE ("Open Camera")) -> (error out=w426:errorcluster)  [unwired: 1 in, 1 out]
            n158 = property on="Binning" class="Clust (strict)"("DisabledEnum"=w428) -> ("Value"=w487:T4)  [unwired: 2 in, 2 out]
            n159 = property on="Region of Interest" class="Clust (strict)"("DisabledEnum"=w428) -> ("Value"=w486:T3)  [unwired: 2 in, 2 out]
            n160 = control-ref of="Frame Number"() -> (w470:refnum<vi>)
            n161 = control-ref of="Camera Image"() -> (w469:refnum<vi>)
            n162 = property on="Image Type" class="Enum (strict)"() -> ("Value"=w439:T7)  [unwired: 2 in, 2 out]
            n163 = property on="Data Rate" class="Clust (strict)"("DisabledEnum"=w428) -> ("Value"=w483:cluster{"DataRate":T5, "Taps":T6})  [unwired: 2 in, 2 out]
            n164 = call-poly "Set Parameters.vi"("error in (no error)"=w426, "Region of Interest"=w486, "Binning"=w487, "Thorlabs.TSI.TLCameraInterfaces.ITLCamera"=w473) -> ("error out"=w482:errorcluster, "Thorlabs.TSI.TLCameraInterfaces.ITLCamera"=w485:refnum<k24>)  [unwired: 6 in]
            n165 = property on="Frames per Trigger\n(zero for unlimited)" class="DigNum (strict)"() -> ("Value"=w484:u32)  [unwired: 2 in, 2 out]
            n166 = Unbundle By Name(w483) -> ("DataRate"=w432:T5, "Taps"=w445:T6)
            n167 = call-poly "Set Parameters.vi"("error in (no error)"=w482, "FramesPerTrigger_zeroForUnlimited"=w484, "Thorlabs.TSI.TLCameraInterfaces.ITLCamera"=w485) -> ("error out"=w436:errorcluster, "Thorlabs.TSI.TLCameraInterfaces.ITLCamera"=w435:refnum<k24>)  [unwired: 7 in]
            n168 = vi-ref "OnImageFrameAvailable Event Callback - TLCamera Main Color.vi"() -> ("vi reference"=w437:refnum<vi>)
            n169 = call "Get Is DataRate Supported.vi"("error in (no error)"=w436, "Data Rate"=w432, "Thorlabs.TSI.TLCameraInterfaces.ITLCamera"=w435) -> ("error out"=w433:errorcluster, "Is DataRate Supported"=w431:bool, "Thorlabs.TSI.TLCameraInterfaces.ITLCamera"=w434:refnum<k24>)  [unwired: 6 in]
            n170 = case shown="True" w431 {
              tunnel: [w489 w495] -> w450
              tunnel: [w490 w494] -> w449
              tunnel: w434 -> [w490 w493]
              tunnel: w433 -> [w489 w492]
              tunnel: w432 -> [_ w491]
              frame False {
              }
              frame True {
                n171 = call-poly "Set Parameters.vi"("error in (no error)"=w492, "DataRate"=w491, "Thorlabs.TSI.TLCameraInterfaces.ITLCamera"=w493) -> ("error out"=w495:errorcluster, "Thorlabs.TSI.TLCameraInterfaces.ITLCamera"=w494:refnum<k24>)  [unwired: 7 in]
              }
            }
            n172 = call "Get Is Taps Supported.vi"("error in (no error)"=w450, "Taps"=w445, "Thorlabs.TSI.TLCameraInterfaces.ITLCamera"=w449) -> ("error out"=w448:errorcluster, "Is Taps Supported"=w447:bool, "Thorlabs.TSI.TLCameraInterfaces.ITLCamera"=w446:refnum<k24>)  [unwired: 6 in]
            n173 = property on="Trigger Settings" class="Clust (strict)"("DisabledEnum"=w428) -> ("Value"=w481:T8)  [unwired: 2 in, 2 out]
            n174 = case shown="True" w447 {
              tunnel: [w497 w502] -> w441
              tunnel: [w496 w501] -> w440
              tunnel: w448 -> [w496 w499]
              tunnel: w446 -> [w497 w500]
              tunnel: w445 -> [_ w498]
              frame False {
              }
              frame True {
                n175 = call-poly "Set Parameters.vi"("error in (no error)"=w499, "Taps"=w498, "Thorlabs.TSI.TLCameraInterfaces.ITLCamera"=w500) -> ("error out"=w501:errorcluster, "Thorlabs.TSI.TLCameraInterfaces.ITLCamera"=w502:refnum<k24>)  [unwired: 7 in]
              }
            }
            n176 = call "Set Trigger Settings.vi"("error in (no error)"=w440, "Trigger Settings"=w481, "Thorlabs.TSI.TLCameraInterfaces.ITLCamera"=w441) -> ("error out"=w466:errorcluster, "Thorlabs.TSI.TLCameraInterfaces.ITLCamera"=w465:refnum<k24>)  [unwired: 7 in]
            n177 = property on="Exposure (ms)" class="DigNum (strict)"() -> ("Value"=w444:dbl)  [unwired: 2 in, 2 out]
            n178 = Multiply(x=w444, y=1000.0) -> (x*y=w442:dbl)
            n179 = call-poly "Set Parameters.vi"("error in (no error)"=w466, "ExposureTime_us"=w442, "Thorlabs.TSI.TLCameraInterfaces.ITLCamera"=w465) -> ("error out"=w463:errorcluster, "Thorlabs.TSI.TLCameraInterfaces.ITLCamera"=w464:refnum<k24>)  [unwired: 7 in]
            n180 = property on="Black Level" class="DigNum (strict)"() -> ("Value"=w459:u32)  [unwired: 2 in, 2 out]
            n181 = call "Get Is BlackLevel Supported.vi"("error in (no error)"=w463, "Thorlabs.TSI.TLCameraInterfaces.ITLCamera"=w464) -> ("error out"=w460:errorcluster, "Is BlackLevel Supported?"=w462:bool, "Thorlabs.TSI.TLCameraInterfaces.ITLCamera"=w461:refnum<k24>)  [unwired: 7 in]
            n182 = case shown="True" w462 {
              tunnel: w461 -> [w511 w516]
              tunnel: w460 -> [w510 w515]
              tunnel: [w510 w514] -> w458
              tunnel: [w511 w513] -> w457
              tunnel: w459 -> [_ w512]
              frame False {
              }
              frame True {
                n183 = call-poly "Set Parameters.vi"("error in (no error)"=w515, "BlackLevel"=w512, "Thorlabs.TSI.TLCameraInterfaces.ITLCamera"=w516) -> ("error out"=w514:errorcluster, "Thorlabs.TSI.TLCameraInterfaces.ITLCamera"=w513:refnum<k24>)  [unwired: 7 in]
              }
            }
            n184 = property on="Image Type" class="Enum (strict)"("DisabledEnum"=w428) -> ()  [unwired: 2 in, 2 out]
            n185 = property on="Frame Settings" class="Clust (strict)"("DisabledEnum"=w428) -> ()  [unwired: 2 in, 2 out]
            n186 = Unbundle By Name(w481) -> ("Trigger Mode"=w480:T9)
            n187 = property on="Gain" class="DigNum (strict)"() -> ("Value"=w453:u32)  [unwired: 2 in, 2 out]
            n188 = call "Get Is Gain Supported.vi"("error in (no error)"=w458, "Thorlabs.TSI.TLCameraInterfaces.ITLCamera"=w457) -> ("error out"=w455:errorcluster, "Is Gain Supported?"=w454:bool, "Thorlabs.TSI.TLCameraInterfaces.ITLCamera"=w456:refnum<k24>)  [unwired: 7 in]
            n189 = case shown="True" w454 {
              tunnel: w456 -> [w504 w509]
              tunnel: w455 -> [w503 w508]
              tunnel: [w503 w507] -> w452
              tunnel: [w504 w506] -> w451
              tunnel: w453 -> [_ w505]
              frame False {
              }
              frame True {
                n190 = call-poly "Set Parameters.vi"("error in (no error)"=w508, "Gain"=w505, "Thorlabs.TSI.TLCameraInterfaces.ITLCamera"=w509) -> ("error out"=w507:errorcluster, "Thorlabs.TSI.TLCameraInterfaces.ITLCamera"=w506:refnum<k24>)  [unwired: 7 in]
              }
            }
            n191 = Bundle("Thorlabs.TSI.TLCameraInterfaces.ITLCamera"=w451, "Frame Number"=w470, "Camera Image"=w469, "Value"=w439, "Color Processor References"=w438) -> (w468:T14)  [unwired: 1 in]
            n192 = node(w452, w451, w437, w468) -> (→"event callback refnum":refnum<k27>, w471:errorcluster)  [unwired: 1 in]
            n193 = call "Arm TLCamera.vi"("error in (no error)"=w471, "Thorlabs.TSI.TLCameraInterfaces.ITLCamera"=w451) -> ("error out"=w476:errorcluster, "Thorlabs.TSI.TLCameraInterfaces.ITLCamera"=w477:refnum<k24>)  [unwired: 8 in]
            n194 = Equal?(x=w480, y=Trigger_Modes."Software") -> (x = y?=w478:bool)
            n195 = case shown="True" w478 {
              tunnel: w477 -> [w518 w522]
              tunnel: w476 -> [w517 w521]
              tunnel: [w518 w520] -> w475
              tunnel: [w517 w519] -> w430
              frame False {
              }
              frame True {
                n196 = call "Issue Software Trigger.vi"("error in (no error)"=w521, "Thorlabs.TSI.TLCameraInterfaces.ITLCamera"=w522) -> ("error out"=w519:errorcluster, "Thorlabs.TSI.TLCameraInterfaces.ITLCamera"=w520:refnum<k24>)  [unwired: 8 in]
              }
            }
            n197 = property on="Stop Camera" class="Bool (strict)"(error in=w430, "DisabledEnum"=T13."Enabled" ("Disabled")) -> (error out=w472:errorcluster)  [unwired: 1 in, 1 out]
          }
          event "Stop Camera": Value Change {
            n198 = event-data() -> ("NewVal"=w524:bool)  [unwired: 1 in, 5 out]
            n199 = case shown="True" w524 {
              tunnel: w529 -> [w530 w549]
              tunnel: [w531 w539] -> w528
              tunnel: [w530 w538] -> w527
              tunnel: w525 -> [w531 w537]
              frame False {
              }
              frame True {
                w543 = T13."Enabled" ("Disabled")
                n200 = property on="event callback refnum" class="Ref (strict)"() -> ("Value"=w534:refnum<k27>)  [unwired: 2 in, 2 out]
                n201 = Not A Number/Path/Refnum?(number/path/refnum=w534) -> (NaN/Path/Refnum?=w536:bool)
                n202 = call "Disarm TLCamera.vi"("error in (no error)"=w549, "Thorlabs.TSI.TLCameraInterfaces.ITLCamera"=w537) -> ("error out"=w535:errorcluster, "Thorlabs.TSI.TLCameraInterfaces.ITLCamera"=w539:refnum<k24>)  [unwired: 8 in]
                n203 = case shown="False" w536 {
                  tunnel: w535 -> [w551 w553]
                  tunnel: w534 -> [w552 _]
                  tunnel: [w550 w553] -> w533
                  frame False {
                    n204 = Unregister For Events(event registration refnum=w552, error in=w551) -> (error out=w550:errorcluster)
                  }
                  frame True {
                  }
                }
                n205 = property on="Data Rate" class="Clust (strict)"(error in=w533, "DisabledEnum"=w543) -> (error out=w548:errorcluster)  [unwired: 1 in, 1 out]
                n206 = property on="Frame Settings" class="Clust (strict)"(error in=w548, "DisabledEnum"=w543) -> (error out=w547:errorcluster)  [unwired: 1 in, 1 out]
                n207 = property on="Image Type" class="Enum (strict)"() -> ("Value"=w532:T7)  [unwired: 2 in, 2 out]
                n208 = property on="Image Type" class="Enum (strict)"(error in=w547, "DisabledEnum"=w543, "Val(Sgnl)"=w532) -> (error out=w546:errorcluster)  [unwired: 1 in, 1 out]
                n209 = property on="Region of Interest" class="Clust (strict)"(error in=w546, "DisabledEnum"=w543) -> (error out=w545:errorcluster)  [unwired: 1 in, 1 out]
                n210 = property on="Trigger Settings" class="Clust (strict)"(error in=w545, "DisabledEnum"=w543) -> (error out=w544:errorcluster)  [unwired: 1 in, 1 out]
                n211 = property on="Start Camera" class="Bool (strict)"(error in=w544, "DisabledEnum"=w543) -> (error out=w542:errorcluster)  [unwired: 1 in, 1 out]
                n212 = property on="Stop Camera" class="Bool (strict)"(error in=w542, "DisabledEnum"=T13."Disabled and Grayed Out" ("Disabled"), "Value"=FALSE ("Stop Camera")) -> (error out=w538:errorcluster)  [unwired: 1 in, 1 out]
              }
            }
          }
        }
        n213 = Unbundle By Name(w62) -> ("status"=w61:bool)
        n214 = case shown="False" w61 {
          tunnel: w60 -> [w69 _]
          tunnel: [w69 Status_-_Main."Close"] -> w59
          frame False {
          }
          frame True {
          }
        }
      }
      frame "Close" {
        w571 = T13."Disabled and Grayed Out" ("Disabled")
        n215 = call <vilib>:"Simple Error Handler.vi"("error in (no error)"=w563) -> ("error out"=w562:errorcluster)  [unwired: 4 in, 4 out]
        n216 = call <vilib>:"Clear Errors.vi"("error in (no error)"=w562) -> ("error out"=w561:errorcluster)  [unwired: 5 in, 1 out]
        n217 = property on="event callback refnum" class="Ref (strict)"(error in=w561) -> (error out=w565:errorcluster, "Value"=w566:refnum<k27>)  [unwired: 1 in, 1 out]
        n218 = Not A Number/Path/Refnum?(number/path/refnum=w566) -> (NaN/Path/Refnum?=w567:bool)
        n219 = case shown="False" w567 {
          tunnel: w566 -> [w585 _]
          tunnel: w565 -> [w584 w586]
          tunnel: [w583 w586] -> w564
          frame False {
            n220 = Unregister For Events(event registration refnum=w585, error in=w584) -> (error out=w583:errorcluster)
          }
          frame True {
          }
        }
        n221 = Not A Number/Path/Refnum?(number/path/refnum=w577) -> (NaN/Path/Refnum?=w578:bool)
        n222 = case shown="False" w578 {
          tunnel: w577 -> [w589 _]
          tunnel: w564 -> [w588 w590]
          tunnel: [w587 w590] -> w557
          frame False {
            n223 = call "Close TLCamera.vi"("error in (no error)"=w588, "Thorlabs.TSI.TLCameraInterfaces.ITLCamera"=w589) -> ("error out"=w587:errorcluster)  [unwired: 9 in]
          }
          frame True {
          }
        }
        n224 = call "Close Color Processors.vi"("error in (no error)"=w557, "Color Processor References"=w555) -> ("error out"=w556:errorcluster)  [unwired: 9 in]
        n225 = call <vilib>:"Simple Error Handler.vi"("error in (no error)"=w556) -> ("error out"=w560:errorcluster)  [unwired: 4 in, 4 out]
        n226 = call <vilib>:"Clear Errors.vi"("error in (no error)"=w560) -> ("error out"=w559:errorcluster)  [unwired: 5 in, 1 out]
        n227 = call "Close TLCameraSDK.vi"("error in (no error)"=w559, "Thorlabs.TSI.TLCameraInterfaces.ITLCameraSDK"=w582) -> ("error out"=w576:errorcluster)  [unwired: 9 in]
        n228 = property on="Start Camera" class="Bool (strict)"(error in=w576, "DisabledEnum"=w571) -> (error out=w575:errorcluster)  [unwired: 1 in, 1 out]
        n229 = property on="Stop Camera" class="Bool (strict)"(error in=w575, "DisabledEnum"=w571) -> (error out=w574:errorcluster)  [unwired: 1 in, 1 out]
        n230 = property on="Open Camera" class="Bool (strict)"(error in=w574, "DisabledEnum"=w571) -> (error out=w573:errorcluster)  [unwired: 1 in, 1 out]
        n231 = property on="Close Camera" class="Bool (strict)"(error in=w573, "DisabledEnum"=w571) -> (error out=w572:errorcluster)  [unwired: 1 in, 1 out]
        n232 = property on="Camera Settings" class="Clust (strict)"(error in=w572, "DisabledEnum"=w571) -> (error out=w570:errorcluster)  [unwired: 1 in, 1 out]
        n233 = property on="Refresh" class="Bool (strict)"(error in=w570, "DisabledEnum"=T13."Enabled" ("Disabled")) -> (error out=w569:errorcluster)  [unwired: 1 in, 1 out]
        n234 = property on="Exit" class="Bool (strict)"(error in=w569, "Value"=FALSE ("Exit")) -> (error out=w558:errorcluster)  [unwired: 1 in, 1 out]
      }
    }
    "Status" <- w7
  }
  n235 = for {
    N: 1 -> [_]
  }
  n236 = call <vilib>:"Simple Error Handler.vi"("error in (no error)"=w2) -> ()  [unwired: 4 in, 5 out]
